vi "RunTestsforEXE.vi"(8 "error in (no error)":errorcluster, 10 "Drona Tests PPL":path=path "D:/Github/solitontech/SLL-Drona/src/example/SimpleCalculator/builds/Tests/SimpleCalculatorDronaTests.lvlibp", 11 "EXE Path":path=path "D:/Github/solitontech/SLL-Drona/src/example/SimpleCalculator/builds/SimpleCalculator.exe") -> (0 "error out":errorcluster)   [LabVIEW 2016, in "Drona.lvlib"]
uses:
  Drona.lvlib
  Setup/GetVI/GetVIByPath.vi
  Stimulus/VI/RunVI.vi
  Setup/GetVI/GetVI.lvlib
  Stimulus/VI/VI.lvlib
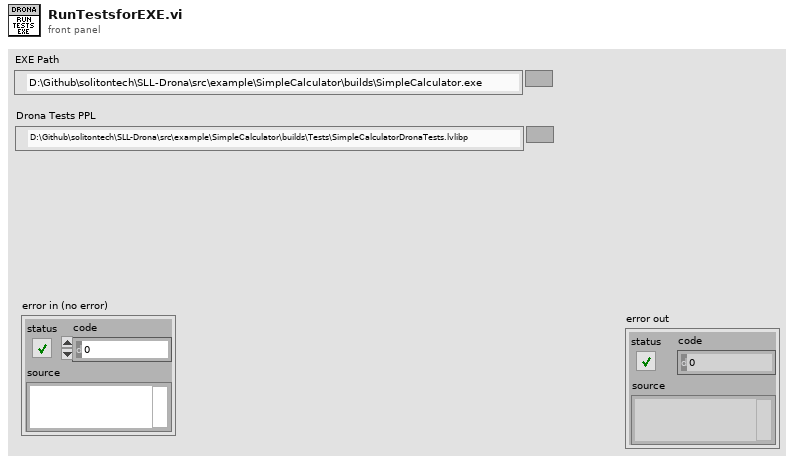
[diagram p1: front panel]
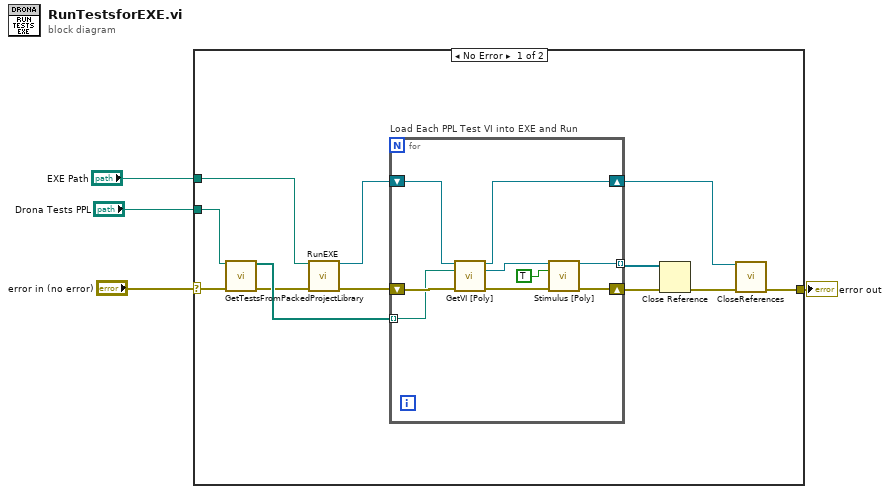
[diagram p0: block diagram]
diagram:
  n1 = case shown="No Error" "error in (no error)" {
    selector: "error in (no error)" -> [w8 w26]
    tunnel: "Drona Tests PPL" -> [w16 _]
    tunnel: "EXE Path" -> [w10 _]
    tunnel: [w9 w26] -> w2
    frame No Error {
      n2 = call "GetTestsFromPackedProjectLibrary.vi"("Packed Project Library Path"=w16, "error in (no error)"=w8) -> ("Tests"=w14:path[], "error out"=w11:errorcluster)  [unwired: 12 in]
      n3 = call "RunEXE.vi"("EXE Path"=w10, "error in (no error)"=w11) -> ("Application Ref"=w7:refnum<vi>, "error out"=w12:errorcluster)  [unwired: 12 in]
      n4 = for "Load Each PPL Test VI into EXE and Run" {
        shift-right: [w22] -> w15
        shift-left: w12 -> [w21]
        tunnel: w14 -> [w20] mode=indexing
        shift-right: [w19] -> w13
        shift-left: w7 -> [w25]
        tunnel: [w17] -> w5 mode=indexing
        n5 = call-poly "GetVI [Poly].vi"("Application Ref in"=w25, "VI Path"=w20, "error in (no error)"=w21) -> ("Application Ref out"=w19:refnum<vi>, "VI Reference"=w24:refnum<vi>, "error out"=w23:errorcluster)  [unwired: 10 in]
        n6 = call-poly "Stimulus [Poly].vi"("VI Reference In"=w24, "Wait Until Done (F)"=TRUE, "error in"=w23) -> ("VI Reference Out"=w17:refnum<vi>, "error out"=w22:errorcluster)  [unwired: 11 in]
      }
      n7 = Close Reference(reference=w5, error in (no error)=w15) -> (error out=w6:errorcluster)
      n8 = call "CloseReferences.vi"("Application Ref"=w13, "error in"=w6) -> ("error out"=w9:errorcluster)  [unwired: 13 in]
    }
    frame Error {
    }
  }
  "error out" <- w2
